vi "https.post.vi"(6 "specific headers in":cluster{"header":T1, "value":string}[](array[cluster]), 8 "error in":errorcluster, 9 "Request body":string, 10 "Path":string, 11 "Nominal Client in":refnum<class "Nominal Client.lvclass">) -> (0 "error out":errorcluster, 2 "Response":string, 3 "Nominal Client out":refnum<class "Nominal Client.lvclass">, 4 "Response Headers":refnum<class "Response Headers.lvclass">)   [LabVIEW 2020, in "Nominal Client.lvclass"]
uses:
  Nominal Client.lvclass
  <vilib>/NI/Advanced HTTP Client/Header--Combo Box.ctl
  <vilib>/addons/_JKI.lib/REST Client/classes/Response Headers/Response Headers.lvclass
  Nominal Client.lvclass/Nominal Client.ctl
  <vilib>/addons/_JKI.lib/REST Client/classes/REST Client/REST Client.lvclass
  <vilib>/NI/Advanced HTTP Client/Session.lvclass
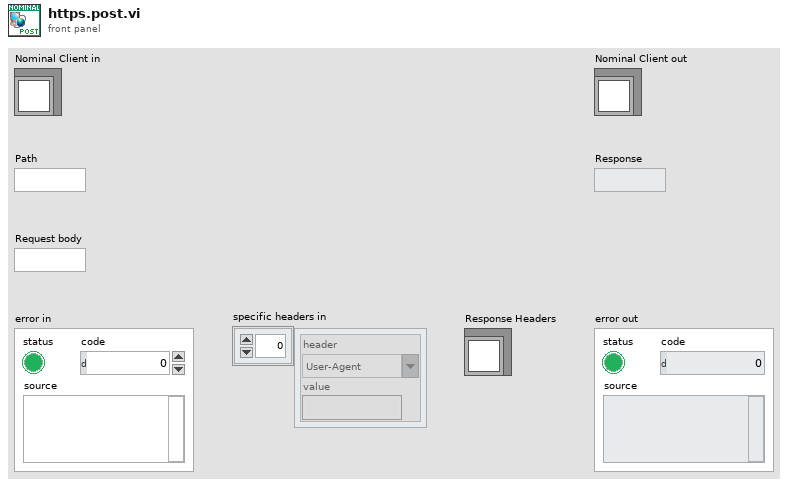
[diagram p1: front panel]
types:
  T1 = typedef "lib_NI_Advanced HTTP Client.lvlib/Session.lvclass/Header--Combo Box.ctl" = string
  T2 = typedef "Nominal Client.lvclass/private_data.ctl" = cluster{"API Token":string, "REST Client":refnum<class "REST Client.lvclass">}
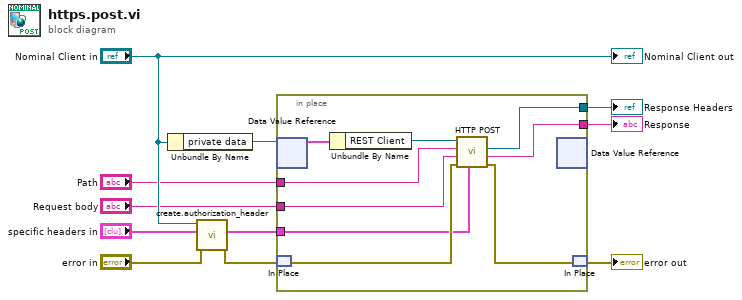
[diagram p0: block diagram]
diagram:
  n1 = Unbundle By Name("Nominal Client in") -> ("private data"=w9:refnum<data-value>)
  n2 = call "create.authorization_header.vi"("error in"="error in", "specific headers in"="specific headers in", "Nominal Client in"="Nominal Client in") -> ("error out"=w4:errorcluster, "specific headers out"=w10:cluster{"header":T1, "value":string}[])  [unwired: 6 in, 1 out]
  n3 = in-place {
    in-place-border: w10 -> [w13]
    in-place-border: [w16] -> w2
    in-place-border: [w17] -> w3
    in-place-border: "Path" -> [w18]
    in-place-border: "Request body" -> [w12]
    n4 = in-place-dvr #1(w9) -> (w20:T2)  [unwired: 1 out]
    n5 = in-place-match #2(w4) -> (w14:errorcluster)
    n6 = Unbundle By Name(w20) -> ("REST Client"=w19:refnum<class "REST Client.lvclass">)
    n7 = call-dynamic "HTTP POST.vi"("request specific headers"=w13, "error in (no error)"=w14, "Request body"=w12, "Path"=w18, "REST Client in"=w19) -> ("error out"=w15:errorcluster, "Response body"=w16:string, "Response Headers"=w17:refnum<class "Response Headers.lvclass">)  [unwired: 1 in, 3 out]
    n8 = in-place-dvr #1() -> ()  [unwired: 1 in, 2 out]
    n9 = in-place-match #2(w15) -> (→"error out":errorcluster)
  }
  "Response Headers" <- w3
  "Response" <- w2
  "Nominal Client out" <- "Nominal Client in"
